vi "Barcode Reader.vi"() -> ()   [LabVIEW 2017]
uses:
  <vilib>/userdefined/High Color/IMAQdx.ctl
  <vilib>/vision/driver/NI_Vision_Acquisition_Software.lvlib
  <vilib>/vision/NI_Vision_Development_Module.lvlib
panel:
  out "Found":bool
  out "error out 3":errorcluster
  out "Data":string
  in  "Barcode Types To Search":u32[](array[ring])=[6, 4] items=["Reserved", "Codabar", "Code 39", "Code 93", "Code 128", "EAN 8", "EAN 13", "Interleaved 2 of 5", "MSI", "UPCA", "Pharmacode", "RSS Limited"]
  in  "stop":bool
  out "error out 2":errorcluster
  out "error out":errorcluster
  in  "Session In":T1
  out "Image":T2(plugin-control)
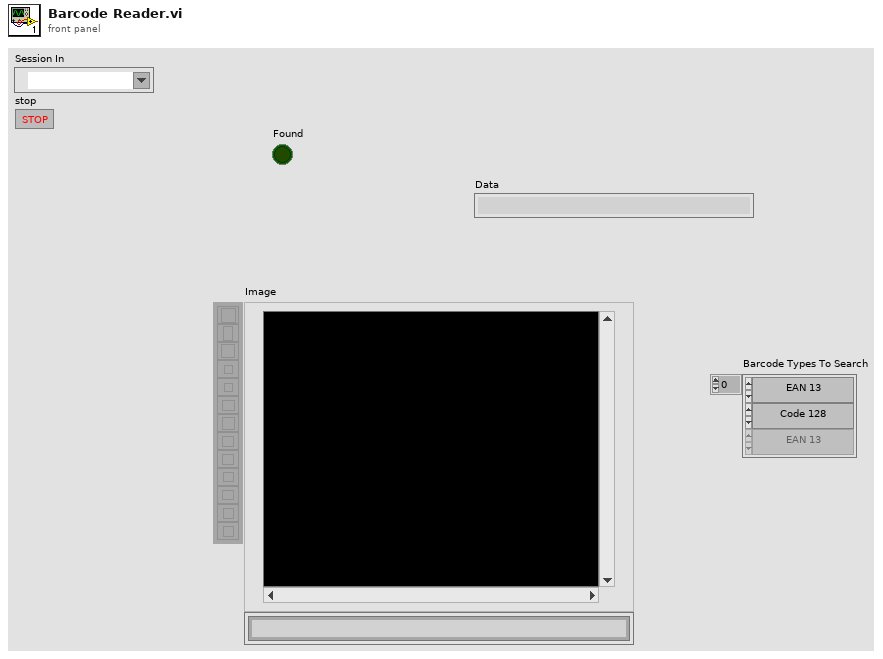
[diagram p1: front panel]
types:
  T1 = typedef "IMAQdx.ctl" = refnum<k21>
  T2 = typedef "IMAQ Image.ctl" = refnum<image>
  T3 = typedef "Image Type" = u32
  T4 = cluster{"Data":string, "Special Char 1":string, "Special Char 2":string, "Checksum(s)":string, "Barcode Type":u32, "Confidence Level":sgl, "Bounding Box":cluster{"x":sgl, "y":sgl}[]}[]
  T5 = cluster{"Data":string, "Special Char 1":string, "Special Char 2":string, "Checksum(s)":string, "Barcode Type":u32, "Confidence Level":sgl, "Bounding Box":cluster{"x":sgl, "y":sgl}[]}
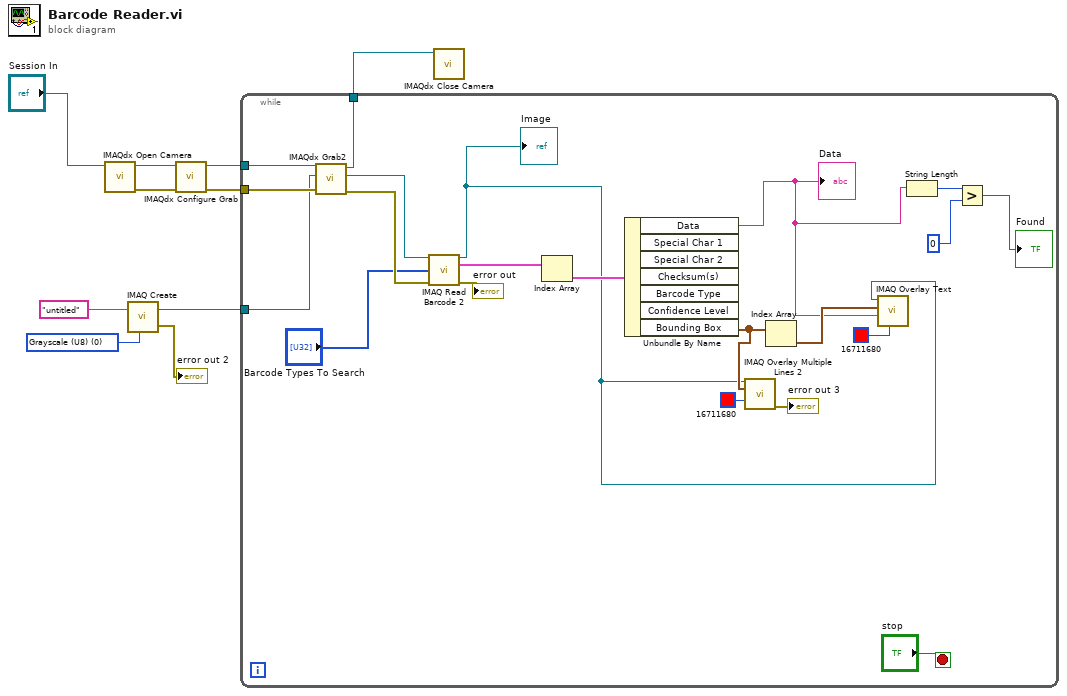
[diagram p0: block diagram]
diagram:
  w2 = T3 0 items=["Grayscale (U8)", "Grayscale (I16)", "Grayscale (SGL)", "Complex (CSG)", "RGB (U32)", "HSL (U32)", "RGB (U64)", "Grayscale (U16)"] ("Image Type")
  n1 = call <vilib>:"IMAQdx Open Camera.vi"("Session In"="Session In") -> ("error out"=w9:errorcluster, "Session Out"=w10:T1)  [unwired: 9 in]
  n2 = call "IMAQ Create"("Image Name"="untitled", "Image Type"=w2) -> ("New Image"=w3:T2, "error out"=→"error out 2":errorcluster)  [unwired: 3 in]
  n3 = call <vilib>:"IMAQdx Configure Grab.vi"("error in"=w9, "Session In"=w10) -> ("error out"=w4:errorcluster, "Session Out"=w6:T1)  [unwired: 8 in]
  n4 = while {
    tunnel: w6 -> [w31]
    tunnel: [w30] -> w5
    tunnel: w4 -> [w29]
    tunnel: w3 -> [w28]
    stop <- "stop" stop-if-true
    n5 = call <vilib>:"IMAQdx Grab2.vi"("error in"=w29, "Image In"=w28, "Session In"=w31) -> ("error out"=w27:errorcluster, "Image Out"=w12:T2, "Session Out"=w30:T1)  [unwired: 5 in, 1 out]
    n6 = call "IMAQ Read Barcode 2"("Image"=w12, "Barcode Types To Search"="Barcode Types To Search", "error in (no error)"=w27) -> ("Image (duplicate)"=w11:T2, "Barcodes"=w23:T4, "error out"=→"error out":errorcluster)  [unwired: 8 in, 2 out]
    "Image" <- w11
    n7 = Index Array(array=w23) -> (element=w22:T5)  [unwired: 1 in]
    n8 = Unbundle By Name(w22) -> ("Data"=w16:string, "Bounding Box"=w19:cluster{"x":sgl, "y":sgl}[])  [unwired: 5 out]
    "Data" <- w16
    n9 = call "IMAQ Overlay Multiple Lines 2"("Image"=w11, "Line End Points"=w19, "Color"=u32 16711680) -> ("error out"=→"error out 3":errorcluster)  [unwired: 11 in, 1 out]
    n10 = Index Array(array=w19) -> (element=w21:cluster{"x":sgl, "y":sgl})  [unwired: 1 in]
    n11 = call "IMAQ Overlay Text"("Text Color (black)"=u32 16711680, "String"=w16, "Origin"=w21, "Image"=w11) -> ()  [unwired: 6 in, 2 out]
    n12 = String Length(string=w16) -> (length=w14:i32)
    n13 = Greater?(x=w14, y=0) -> (0:→"Found":bool)
  }
  n14 = call <vilib>:"IMAQdx Close Camera.vi"("Session In"=w5) -> ()  [unwired: 10 in, 1 out]
